vi "I16_Read Index Set.vi"(9 "Default":i16[](array[numeric]), 11 "Indices":i32[](array[numeric])) -> (1 "Values":i16[](array[numeric]))   [LabVIEW 2016, in "CVT.lvlib" / "Current Value Table.lvlib"]
doc: "This VI reads a set of data as defined by the GetIndices function. This VI can provide an order of magnitude increase in performance over a normal index read for sufficiently large data sets."
uses:
  Current Value Table.lvlib
  Type Defs/Memory Commands.ctl
  I16_Memory Block.vi
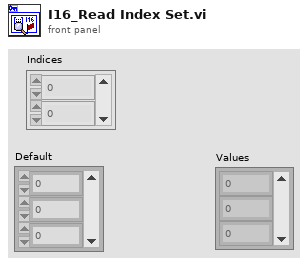
[diagram p1: front panel]
types:
  T1 = typedef "CVT.lvlib/Current Value Table.lvlib/Memory Commands.ctl" = enum16{"Init", "Add Data", "Read", "Read Group", "Read All", "Write", "Write Group", "Get Size"}
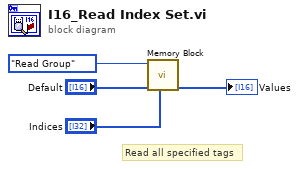
[diagram p0: block diagram]
diagram:
  # "Read all specified tags"
  n1 = call-poly "Memory Block.vi"("Group Indices"="Indices", "Data In"="Default", "Method"=Memory_Commands."Read Group") -> ("Group Data"=→"Values":i16[])  [unwired: 6 in, 2 out]
